vi "Timepos.vi"(3 "error in (no error)":errorcluster, 4 "Numero a colocar":dbl, 5 "Numero a colocar":dbl) -> (0 "error out":errorcluster, 1 "Array 2":dbl[][](array[numeric]), 2 "Array 1":dbl[][](array[numeric]))   [LabVIEW 2016]
panel:
  out "3-4":u32
  out "timer 3":u32
  out "timer 4":u32
  out "timer 1":u32
  out "timer 2":u32
  out "1-2":u32
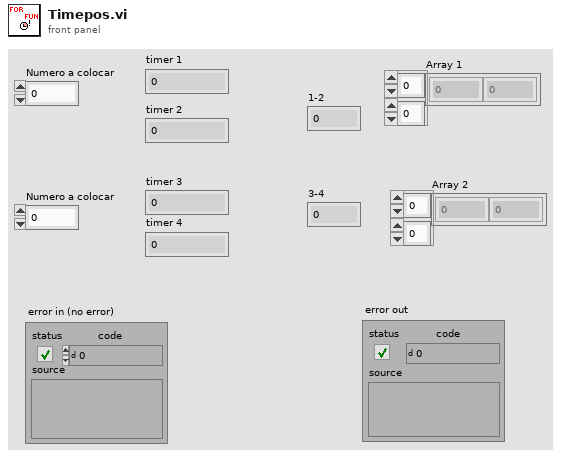
[diagram p1: front panel]
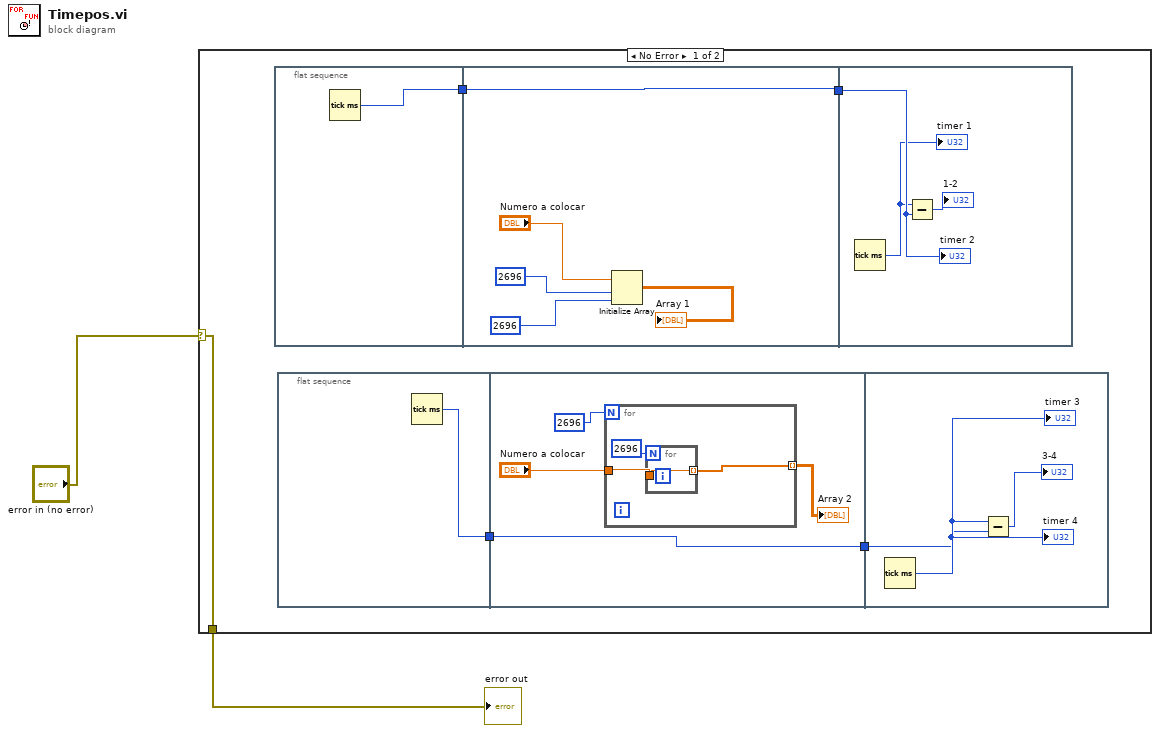
[diagram p0: block diagram]
diagram:
  n1 = case shown="No Error" "error in (no error)" {
    selector: "error in (no error)" -> [w3 w29]
    tunnel: [w3 w29] -> w1
    frame No Error {
      n2 = flat-sequence {
        tunnel: [w20] -> w7
        tunnel: [w21] -> w6
        tunnel: w7 -> [w21]
        tunnel: w6 -> [w28]
        frame #0 {
          n3 = Tick Count (ms)() -> (millisecond timer value=w20:u32)
        }
        frame #1 {
          n4 = Initialize Array("Numero a colocar", 2696 ("dimension size"), 2696 ("dimension size")) -> (→"Array 1":dbl[][])
        }
        frame #2 {
          n5 = Tick Count (ms)() -> (millisecond timer value=w27:u32)
          "timer 1" <- w27
          n6 = Subtract(x=w27, y=w28) -> (x-y=→"1-2":u32)
          "timer 2" <- w28
        }
      }
      n7 = flat-sequence {
        tunnel: [w8] -> w5
        tunnel: [w10] -> w4
        tunnel: w5 -> [w10]
        tunnel: w4 -> [w18]
        frame #0 {
          n8 = Tick Count (ms)() -> (millisecond timer value=w8:u32)
        }
        frame #1 {
          n9 = for {
            N: 2696 -> [_]
            tunnel: [w14] -> w9 mode=indexing
            tunnel: "Numero a colocar" -> [w13]
            n10 = for {
              N: 2696 -> [_]
              tunnel: [w16] -> w14 mode=indexing
              tunnel: w13 -> [w16]
            }
          }
          "Array 2" <- w9
        }
        frame #2 {
          n11 = Tick Count (ms)() -> (millisecond timer value=w19:u32)
          "timer 3" <- w19
          n12 = Subtract(x=w19, y=w18) -> (x-y=→"3-4":u32)
          "timer 4" <- w18
        }
      }
    }
    frame Error {
    }
  }
  "error out" <- w1
